vi "Chirp_WriteFiles.vi"(8 "error in (no error)":errorcluster, 10 "Data":string, 11 "ChirpEIS in":refnum<class "ChirpEIS.lvclass">) -> (0 "error out":errorcluster, 3 "ChirpEIS out":refnum<class "ChirpEIS.lvclass">)   [LabVIEW 2014, in "ChirpEIS.lvclass"]
uses:
  ChirpEIS.lvclass
  ChirpEIS.lvclass/ChirpEIS.ctl
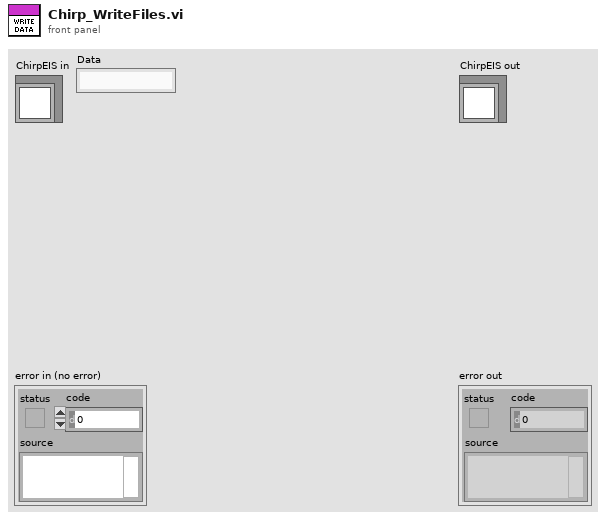
[diagram p1: front panel]
types:
  T1 = enum16{"open", "replace", "create", "open or create", "replace or create", "replace or create with confirmation"}
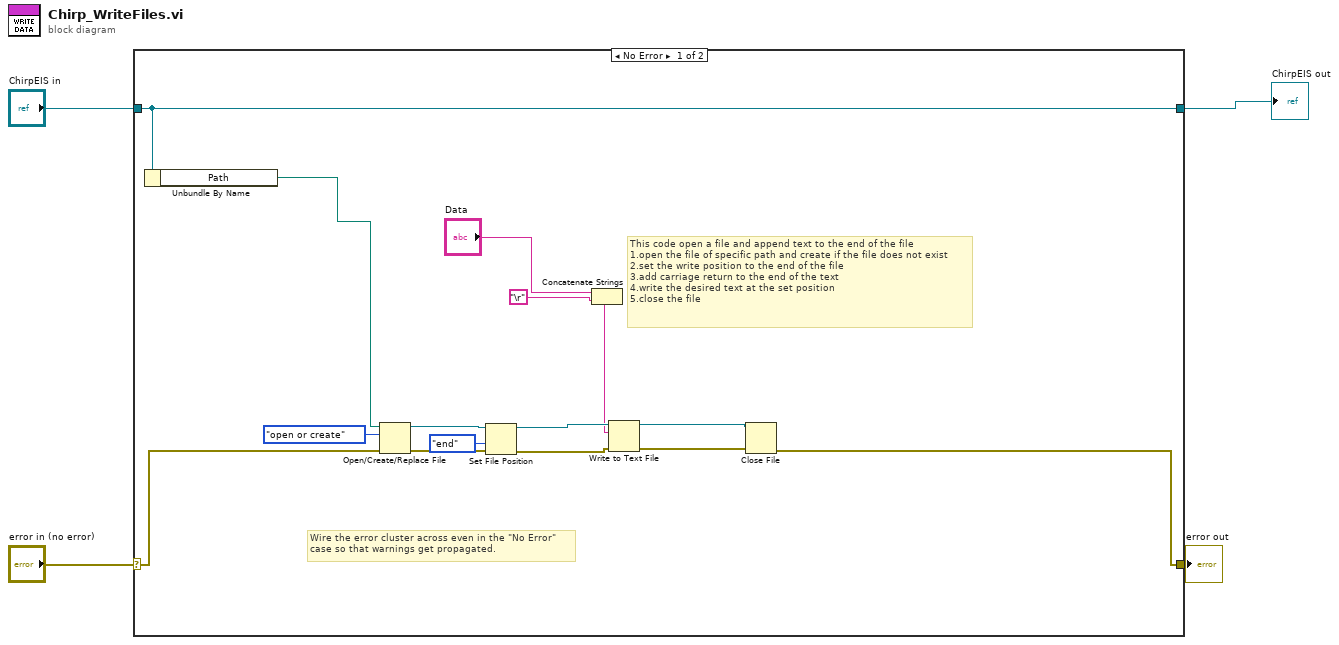
[diagram p0: block diagram]
diagram:
  n1 = case shown="No Error" "error in (no error)" {
    selector: "error in (no error)" -> [w9 w21]
    tunnel: [w8 w21] -> w3
    tunnel: [w7 w20] -> w1
    tunnel: "ChirpEIS in" -> [w7 w20]
    frame No Error {
      # "This code open a file and append text to the end of the file\n1.open the file of specific path and create if the file does not exist\n2.set the write position to the end of the file\n3.add carriage return to the end of the text\n4.write the desired text at the set position\n5.close the file"
      # "Wire the error cluster across even in the \"No Error\"\ncase so that warnings get propagated."
      n2 = Unbundle By Name(w7) -> ("Path"=w6:path)
      n3 = Open/Create/Replace File(file path (use dialog)=w6, error in=w9, operation (0:open)=T1."open or create") -> (refnum out=w18:refnum<file>, error out=w17:errorcluster)  [unwired: 3 in, 1 out]
      n4 = Set File Position(refnum=w18, from (0:start)=enum16{"start", "end", "current"}."end", error in=w17) -> (refnum out=w15:refnum<file>, error out=w14:errorcluster)  [unwired: 1 in]
      n5 = Concatenate Strings("Data", "\r") -> (w10:string)
      n6 = Write to Text File(file (use dialog)=w15, text=w10, error in=w14) -> (refnum out=w13:refnum<file>, error out=w12:errorcluster)  [unwired: 1 in, 1 out]
      n7 = Close File(refnum=w13, error in=w12) -> (error out=w8:errorcluster)  [unwired: 1 out]
    }
    frame Error {
    }
  }
  "error out" <- w3
  "ChirpEIS out" <- w1
